vi "EnFlo_Seeder_Control_Duty_Cycle.vi"(0 "Current Time (s)":dbl) -> ()   [LabVIEW 2013]
panel:
  in  "Sugar Strength":dbl=0.3
  out "Leak Detected":bool
  in  "Performing hand clean":bool
  out "Run Transducer":bool
  out "Sugar Pump":bool
  out "Low Flow":bool
  out "High Flow":bool
  out "Time Since Last Flush (min)":dbl
  out "Running Flush time":dbl
  out "Transducer setting":dbl
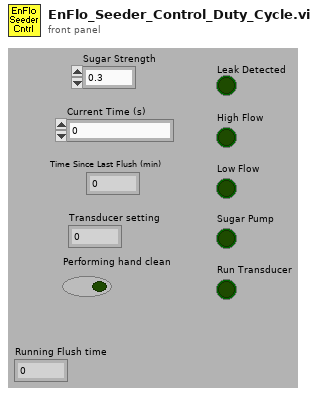
[diagram p1: front panel]
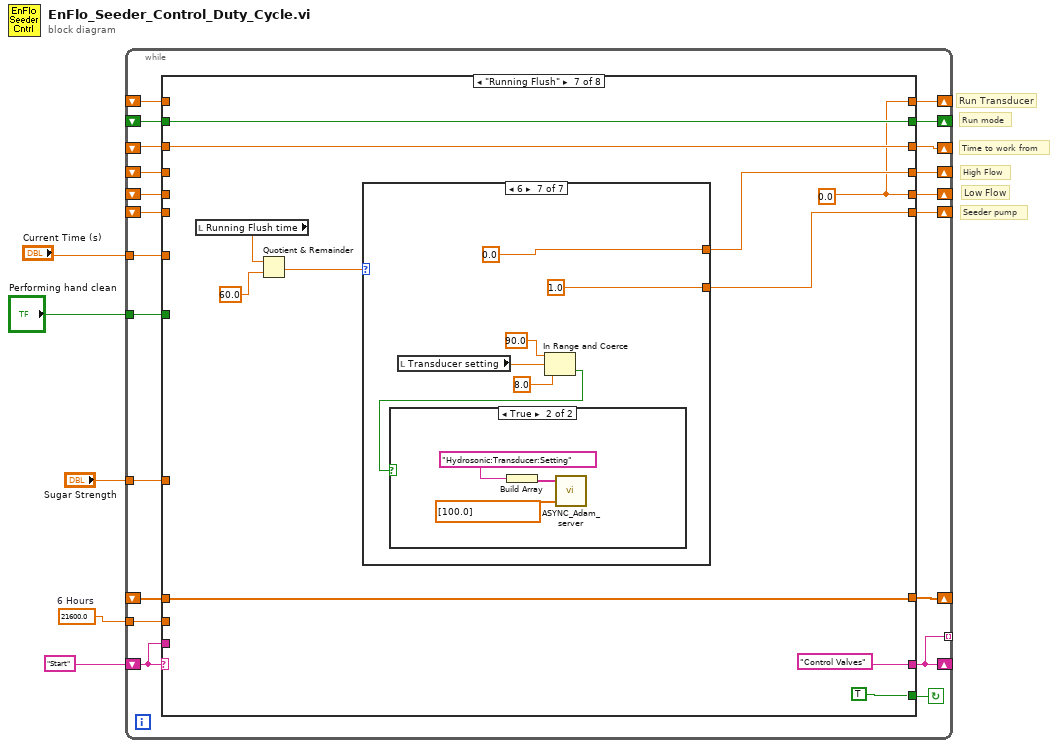
[diagram p0: block diagram]
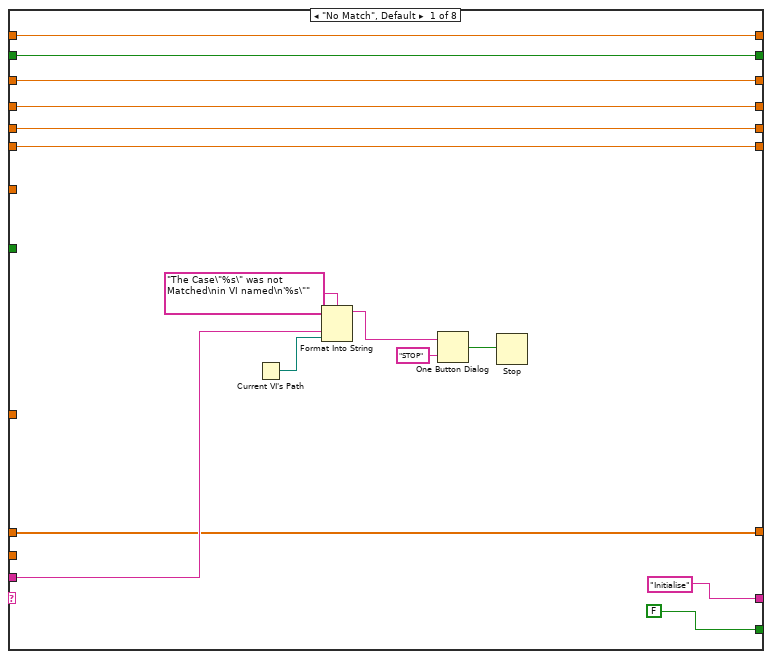
[diagram p2: hidden frame]
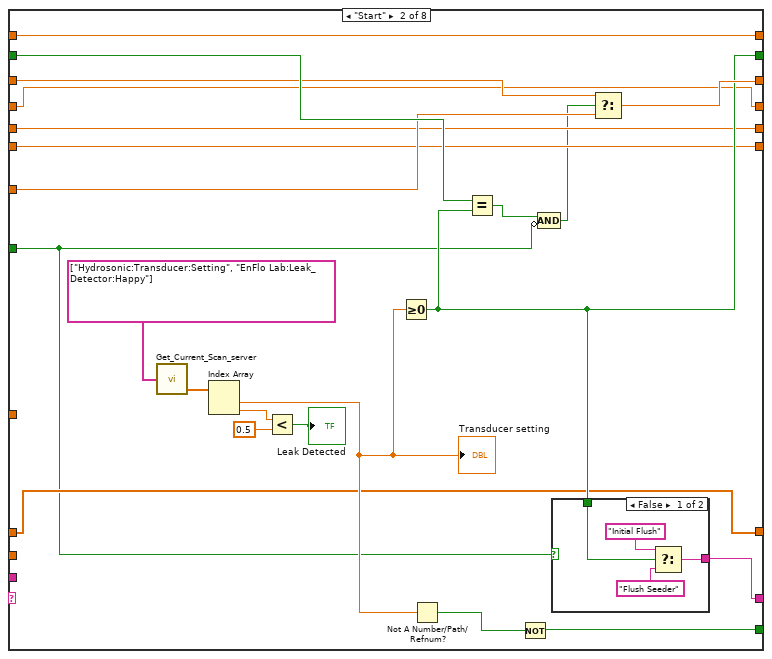
[diagram p3: hidden frame]
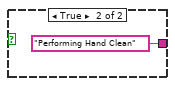
[diagram p4: hidden frame]
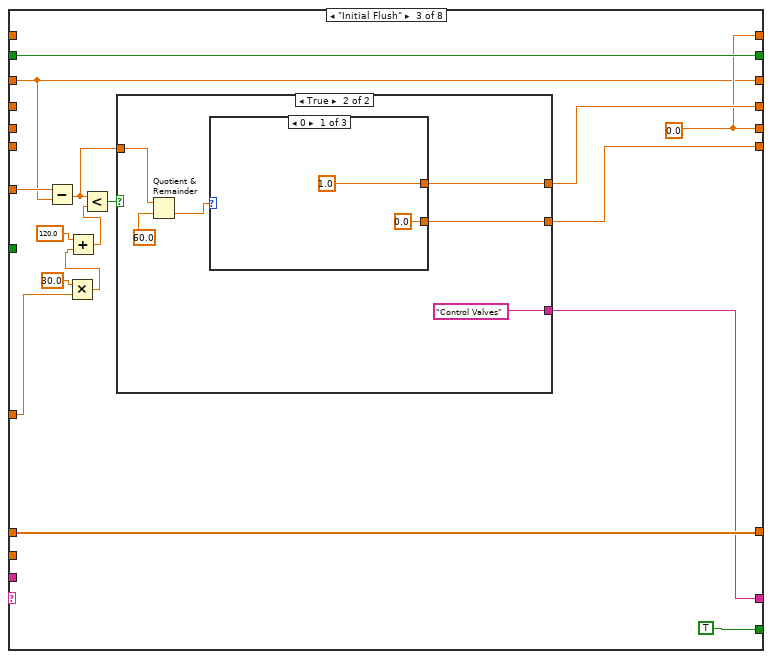
[diagram p5: hidden frame]
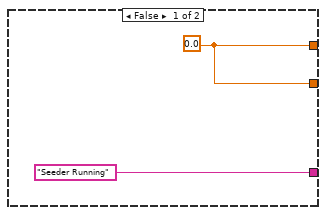
[diagram p6: hidden frame]
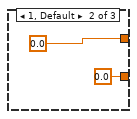
[diagram p7: hidden frame]
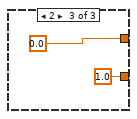
[diagram p8: hidden frame]
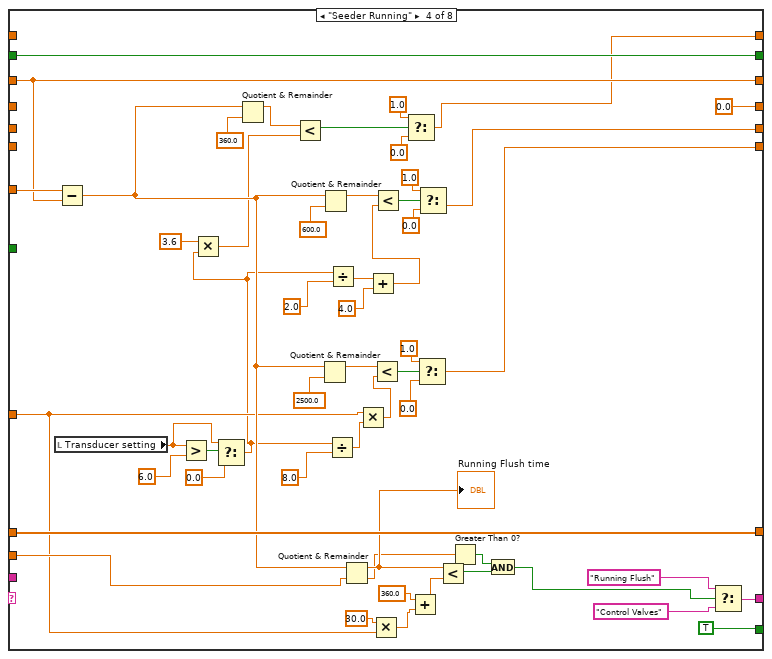
[diagram p9: hidden frame]
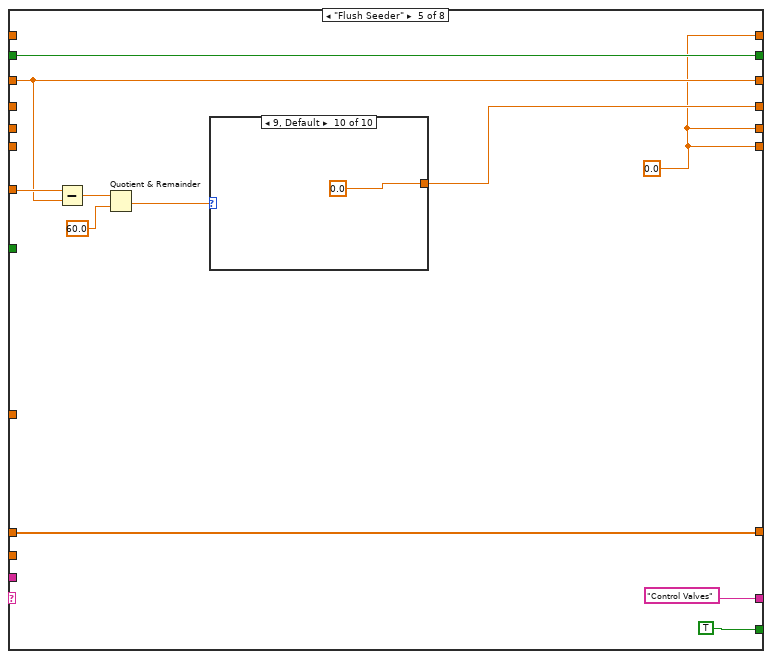
[diagram p10: hidden frame]
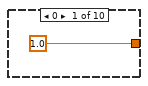
[diagram p11: hidden frame]
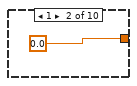
[diagram p12: hidden frame]
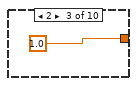
[diagram p13: hidden frame]
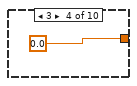
[diagram p14: hidden frame]
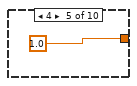
[diagram p15: hidden frame]
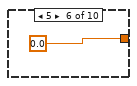
[diagram p16: hidden frame]
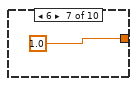
[diagram p17: hidden frame]
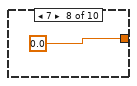
[diagram p18: hidden frame]
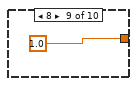
[diagram p19: hidden frame]
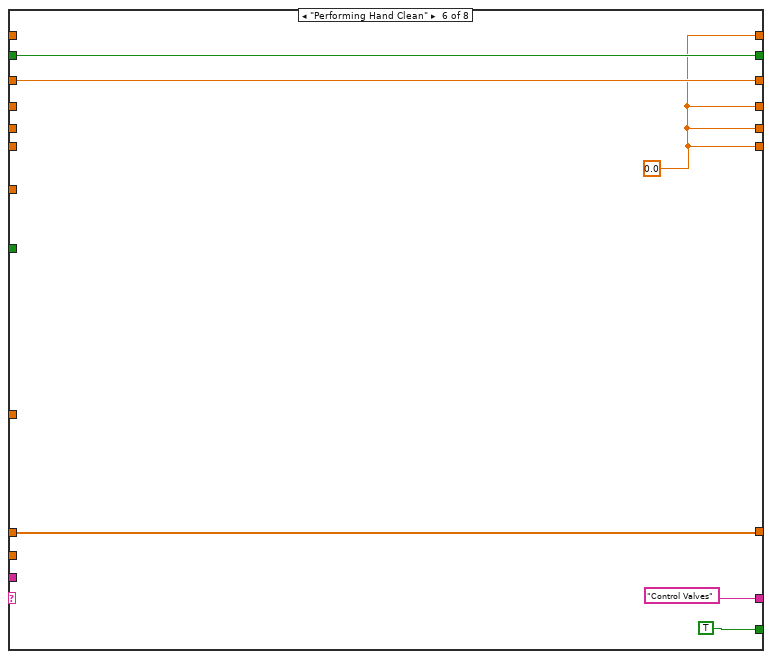
[diagram p20: hidden frame]
diagram:
  w3 = 21600.0  # 6 Hours
  # "Run Transducer"
  # "Seeder pump"
  # "Low Flow"
  # "High Flow"
  # "Run mode"
  # "Time to work from"
  n1 = while {
    shift-left: "Start" -> [w25]
    shift-right: [w9] -> _
    shift-right: [w24] -> _
    shift-left: _ -> [w21]
    shift-right: [w23] -> _
    shift-left: _ -> [w22]
    tunnel: "Current Time (s)" -> [w20]
    shift-right: [w18] -> _
    shift-left: _ -> [w19]
    shift-right: [w17] -> _
    shift-left: _ -> [w16]
    shift-right: [w14] -> _
    shift-left: _ -> [w15]
    shift-right: [w12] -> _
    shift-left: _ -> [w13]
    shift-right: [w11] -> _
    shift-left: _ -> [w10]
    tunnel: [w9] -> _ mode=indexing
    tunnel: w3 -> [w8]
    tunnel: "Performing hand clean" -> [w7]
    tunnel: "Sugar Strength" -> [w6]
    stop <- w26 continue-if-true
    n2 = case shown="\"Running Flush\"" w25 {
      tunnel: [FALSE w61 TRUE TRUE TRUE TRUE TRUE FALSE] -> w26
      tunnel: ["Initialise" w54 w74 w127 "Control Valves" "Control Valves" "Control Valves" "End"] -> w9
      tunnel: w25 -> [w36 _ _ _ _ _ _ _]
      tunnel: [w31 w58 w77 w149 w158 w175 w186 w233] -> w24
      tunnel: [w33 w55 w83 w151 w160 w176 w187 w242] -> w23
      tunnel: w22 -> [w33 w59 w83 w151 w160 w176 w187 w242]
      tunnel: w21 -> [w31 w57 w77 w149 w158 w175 w186 w233]
      tunnel: w20 -> [_ w56 w78 w150 w159 _ _ w234]
      tunnel: w19 -> [w32 w53 _ _ _ _ _ w230]
      tunnel: [w32 w53 w82 0.0 w154 w173 w183 w230] -> w18
      tunnel: w16 -> [w30 w51 _ _ _ _ _ w228]
      tunnel: [w30 w51 w79 w137 w152 w173 w179 w228] -> w17
      tunnel: w15 -> [w29 w50 _ _ _ _ _ w226]
      tunnel: [w29 w50 w80 w130 w152 w173 w180 w226] -> w14
      tunnel: w13 -> [w28 w52 w81 w147 w153 w174 w182 w222]
      tunnel: [w28 w52 w81 w147 w153 w174 w182 w215] -> w12
      tunnel: w10 -> [w27 w49 _ _ _ _ _ w224]
      tunnel: [w27 w49 w79 w117 w152 w173 w179 w224] -> w11
      tunnel: w8 -> [_ _ _ w111 _ _ _ w218]
      tunnel: w7 -> [_ w46 _ _ _ _ _ _]
      tunnel: w6 -> [_ _ w71 w104 _ _ _ _]
      frame "No Match", Default {
        n3 = Current VI's Path() -> (path=w35:path)
        n4 = Format Into String(format string="The Case\"%s\" was not Matched\nin VI named\n'%s\"" ("Format String"), w36, w35) -> (resulting string=w39:string)  [unwired: 2 in, 1 out]
        n5 = One Button Dialog(message=w39, button name ("OK")="STOP") -> (true=w37:bool)
        n6 = Stop(stop? (T)=w37) -> ()
      }
      frame "Start" {
        n7 = call "Get_Current_Scan_server.vi"("Desired Channels"=string[] ["Hydrosonic:Transducer:Setting", "EnFlo Lab:Leak_Detector:Happy"] ("appended array")) -> ("Numerical Values"=w63:dbl[])  [unwired: 2 out]
        n8 = Index Array(array=w63) -> (element #1=w60:dbl, element #2=w44:dbl)  [unwired: 2 in]
        "Transducer setting" <- w60
        n9 = Less?(x=w44, y=0.5) -> (x < y?=→"Leak Detected":bool)
        n10 = Greater Or Equal To 0?(x=w60) -> (x >= 0?=w55:bool)
        n11 = Not A Number/Path/Refnum?(number/path/refnum=w60) -> (NaN/Path/Refnum?=w62:bool)
        n12 = Equal?(x=w59, y=w55) -> (x = y?=w48:bool)
        n13 = Not(x=w62) -> (.not. x?=w61:bool)
        n14 = Compound Arithmetic op=AND(w48, invert w46) -> (w47:bool)
        n15 = case shown="False" w46 {
          tunnel: w55 -> [w67 _]
          tunnel: [w66 "Performing Hand Clean"] -> w54
          frame False {
            n16 = Select(t="Initial Flush", s=w67, f="Flush Seeder") -> (s? t:f=w66:string)
          }
          frame True {
          }
        }
        n17 = Select(t=w57, s=w47, f=w56) -> (s? t:f=w58:dbl)
      }
      frame "Initial Flush" {
        w79 = 0.0
        n18 = Subtract(x=w78, y=w77) -> (x-y=w75:dbl)
        n19 = Multiply(x=30.0 ("y"), y=w71) -> (x*y=w70:dbl)
        n20 = Add(x=120.0 ("y"), y=w70) -> (x+y=w69:dbl)
        n21 = Less?(x=w75, y=w69) -> (x < y?=w76:bool)
        n22 = case shown="True" w76 {
          tunnel: [w86 w92] -> w82
          tunnel: [w86 w91] -> w80
          tunnel: w75 -> [_ w89]
          tunnel: ["Seeder Running" "Control Valves"] -> w74
          frame False {
            w86 = 0.0
          }
          frame True {
            n23 = Quotient & Remainder(x=w89, y=60.0) -> (floor(x/y)=w88:dbl)  [unwired: 1 out]
            n24 = case shown="0" w88 {
              tunnel: [1.0 0.0 0.0] -> w92
              tunnel: [0.0 0.0 1.0] -> w91
              frame 0 {
              }
              frame 1, Default {
              }
              frame 2 {
              }
            }
          }
        }
      }
      frame "Seeder Running" {
        n25 = local read "Transducer setting"() -> (w101:dbl)
        n26 = Subtract(x=w150, y=w149) -> (x-y=w124:dbl)
        n27 = Greater?(x=w101, y=6.0) -> (0:w102:bool)
        n28 = Select(t=w101, s=w102, f=0.0) -> (s? t:f=w99:dbl)
        n29 = Multiply(x=3.6, y=w99) -> (x*y=w121:dbl)
        n30 = Quotient & Remainder(x=w124, y=360.0) -> (x-y*floor(x/y)=w122:dbl)  [unwired: 1 out]
        n31 = Less?(x=w122, y=w121) -> (x < y?=w118:bool)
        n32 = Quotient & Remainder(x=w124, y=2500.0) -> (x-y*floor(x/y)=w132:dbl)  [unwired: 1 out]
        n33 = Quotient & Remainder(x=w124, y=600.0) -> (x-y*floor(x/y)=w146:dbl)  [unwired: 1 out]
        n34 = Divide(x=w99, y=8.0) -> (x/y=w109:dbl)
        n35 = Divide(x=w99, y=2.0) -> (x/y=w142:dbl)
        n36 = Quotient & Remainder(x=w124, y=w111) -> (x-y*floor(x/y)=w126:dbl, floor(x/y)=w115:dbl)
        "Running Flush time" <- w126
        n37 = Multiply(x=w104, y=w109) -> (x*y=w110:dbl)
        n38 = Add(x=w142, y=4.0) -> (x+y=w140:dbl)
        n39 = Multiply(x=30.0 ("y"), y=w104) -> (x*y=w106:dbl)
        n40 = Less?(x=w132, y=w110) -> (x < y?=w133:bool)
        n41 = Less?(x=w146, y=w140) -> (x < y?=w145:bool)
        n42 = Select(t=1.0, s=w118, f=0.0) -> (s? t:f=w117:dbl)
        n43 = Add(x=360.0 ("y"), y=w106) -> (x+y=w105:dbl)
        n44 = Select(t=1.0, s=w133, f=0.0) -> (s? t:f=w130:dbl)
        n45 = Select(t=1.0, s=w145, f=0.0) -> (s? t:f=w137:dbl)
        n46 = Less?(x=w126, y=w105) -> (x < y?=w113:bool)
        n47 = Greater Than 0?(x=w115) -> (x > 0?=w114:bool)
        n48 = And(x=w114, y=w113) -> (x .and. y?=w112:bool)
        n49 = Select(t="Running Flush", s=w112, f="Control Valves") -> (s? t:f=w127:string)
      }
      frame "Flush Seeder" {
        w152 = 0.0
        n50 = Subtract(x=w159, y=w158) -> (x-y=w157:dbl)
        n51 = Quotient & Remainder(x=w157, y=60.0) -> (floor(x/y)=w155:dbl)  [unwired: 1 out]
        n52 = case shown="9, Default" w155 {
          tunnel: [1.0 0.0 1.0 0.0 1.0 0.0 1.0 0.0 1.0 0.0] -> w154
          frame 0 {
          }
          frame 1 {
          }
          frame 2 {
          }
          frame 3 {
          }
          frame 4 {
          }
          frame 5 {
          }
          frame 6 {
          }
          frame 7 {
          }
          frame 8 {
          }
          frame 9, Default {
          }
        }
      }
      frame "Performing Hand Clean" {
        w173 = 0.0
      }
      frame "Running Flush" {
        w179 = 0.0
        n53 = local read "Running Flush time"() -> (w181:dbl)
        n54 = Quotient & Remainder(x=w181, y=60.0) -> (floor(x/y)=w184:dbl)  [unwired: 1 out]
        n55 = case shown="6" w184 {
          tunnel: [1.0 0.0 1.0 0.0 1.0 0.0 0.0] -> w183
          tunnel: [0.0 0.0 0.0 0.0 0.0 0.0 1.0] -> w180
          frame 0 {
          }
          frame 1 {
          }
          frame 2 {
          }
          frame 3 {
          }
          frame 4 {
          }
          frame 5, Default {
          }
          frame 6 {
            n56 = local read "Transducer setting"() -> (w205:dbl)
            n57 = In Range and Coerce(upper limit=90.0, x=w205, lower limit=8.0) -> (In Range?=w202:bool)  [unwired: 1 out]
            n58 = case shown="True" w202 {
              frame False {
              }
              frame True {
                n59 = Build Array("Hydrosonic:Transducer:Setting") -> (w209:string[])
                n60 = call "ASYNC_Adam_server.vi"("Values"=dbl[] [100.0], "Channel Names"=w209) -> ()  [unwired: 1 in, 3 out]
              }
            }
          }
        }
      }
      frame "Control Valves" {
        n61 = Subtract(x=w234, y=w233) -> (x-y=w219:dbl)
        n62 = Quotient & Remainder(x=w219, y=w218) -> (x-y*floor(x/y)=w217:dbl)  [unwired: 1 out]
        n63 = Divide(x=w217, y=60.0) -> (x/y=→"Time Since Last Flush (min)":dbl)
        n64 = Build Array(w224, w230, w228, w226) -> (w212:dbl[])
        n65 = Array Size(array=w222) -> (size(s)=w221:i32)
        n66 = Equal To 0?(x=w221) -> (x = 0?=w220:bool)
        n67 = Array Size(array=w212) -> (size(s)=w214:i32)
        n68 = local read "Leak Detected"() -> (w216:bool)
        n69 = Initialize Array(0.0 ("element"), w214) -> (w211:dbl[])
        n70 = Select(t=w211, s=w216, f=w212) -> (s? t:f=w215:dbl[])
        n71 = case shown="False" w220 {
          tunnel: w215 -> [w247 w252]
          tunnel: string[] ["Hydrosonic:Seeder:Enable", "EnFlo_Tunnel:Seeder:High_Flow", "EnFlo_Tunnel:Seeder:Low_Flow", "EnFlo_Tunnel:Seeder_Pump:Enable"] ("Desired Ch Names") -> [w246 w253]
          tunnel: [w245 w253] -> w238
          tunnel: [w244 w252] -> w237
          tunnel: w222 -> [w243 _]
          frame False {
            n72 = for {
              tunnel: w243 -> [w251] mode=indexing
              tunnel: w247 -> [w250] mode=indexing
              tunnel: [w250] -> w244 mode=indexing if=w248
              tunnel: w246 -> [w249] mode=indexing
              tunnel: [w249] -> w245 mode=indexing if=w248
              n73 = Not Equal?(x=w250, y=w251) -> (x != y?=w248:bool)
            }
          }
          frame True {
          }
        }
        n74 = Array Size(array=w237) -> (size(s)=w241:i32)
        n75 = Greater Than 0?(x=w241) -> (x > 0?=w240:bool)
        n76 = case shown="True" w240 {
          tunnel: w237 -> [_ w255]
          tunnel: w238 -> [_ w254]
          frame False {
          }
          frame True {
            n77 = call "ASYNC_Adam_server.vi"("Values"=w255, "Channel Names"=w254) -> ()  [unwired: 1 in, 3 out]
          }
        }
        n78 = Greater Than 0?(x=w230) -> (x > 0?=→"High Flow":bool)
        n79 = Greater Than 0?(x=w228) -> (x > 0?=→"Low Flow":bool)
        n80 = Greater Than 0?(x=w224) -> (x > 0?=→"Run Transducer":bool)
        n81 = Greater Than 0?(x=w226) -> (x > 0?=→"Sugar Pump":bool)
      }
    }
  }
